vi "Find Project Library.vi"(8 "error in (no error)":errorcluster, 10 "library name":string, 11 "project ref":refnum<vi>) -> (0 "error out":errorcluster, 2 "found?":bool, 3 "library ref":refnum<vi>)   [LabVIEW 2027, in "Build Automation.lvlib"]
uses:
  Build Automation.lvlib
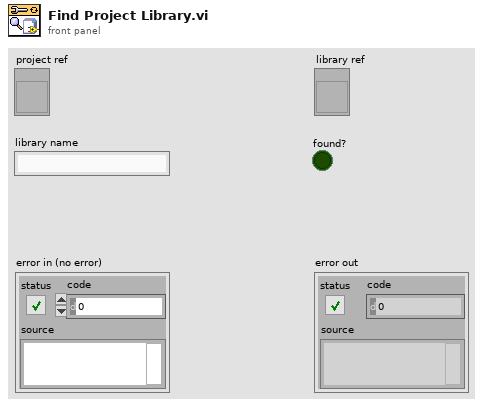
[diagram p1: front panel]
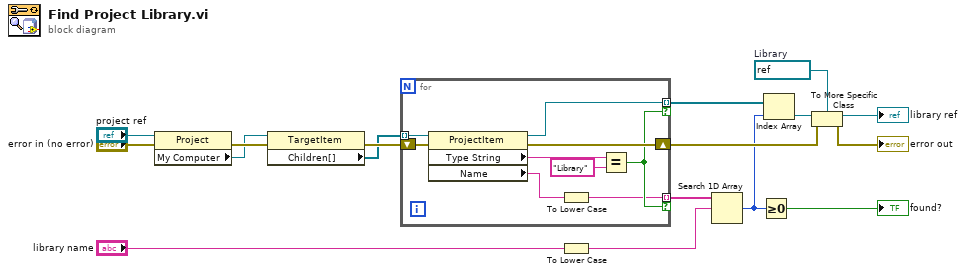
[diagram p0: block diagram]
diagram:
  w8 = refnum<vi> refnum  # Library
  n1 = property class="Project"(reference="project ref", error in="error in (no error)") -> (error out=w17:errorcluster, "My Computer"=w15:refnum<vi>)  [unwired: 1 out]
  n2 = property class="TargetItem"(reference=w15, error in=w17) -> (error out=w16:errorcluster, "Children[]"=w9:refnum<vi>[])  [unwired: 1 out]
  n3 = for {
    tunnel: w9 -> [w26] mode=indexing
    tunnel: [w20] -> w12 mode=indexing if=w19
    tunnel: [w18] -> w14 mode=indexing if=w19
    shift-right: [w22] -> w6
    shift-left: w16 -> [w23]
    n4 = property class="ProjectItem"(reference=w26, error in=w23) -> (reference out=w20:refnum<vi>, error out=w22:errorcluster, "Type String"=w21:string, "Name"=w24:string)
    n5 = To Lower Case(string=w24) -> (all lower case string=w18:string)
    n6 = Equal?(x=w21, y="Library") -> (x = y?=w19:bool)
  }
  n7 = To Lower Case(string="library name") -> (all lower case string=w1:string)
  n8 = Search 1D Array(1D array=w14, element=w1) -> (index of element=w3:i32)  [unwired: 1 in]
  n9 = Greater Or Equal To 0?(x=w3) -> (x >= 0?=→"found?":bool)
  n10 = Index Array(array=w12, index=w3) -> (element=w7:refnum<vi>)
  n11 = To More Specific Class(target class=w8, reference=w7, error in=w6) -> (specific class reference=→"library ref":refnum<vi>, error out=→"error out":errorcluster)
